vi "Arcade Drive.vi"(8 "b":dbl=1.0, 9 "a":dbl=1.0, 11 "Drive Metrics In":T1) -> (3 "Drive Metrics out":T1)   [LabVIEW 2014]
uses:
  Drive Train Metrics.ctl
  CmdFlag.ctl
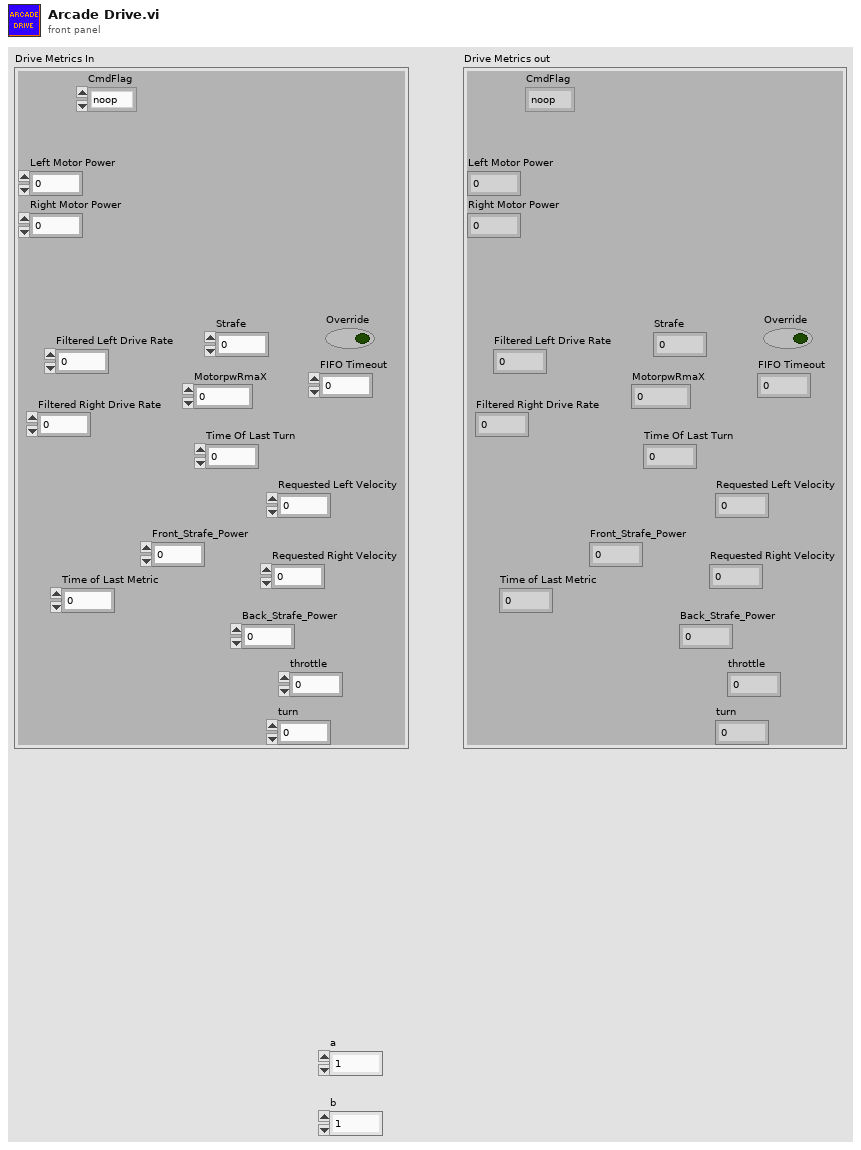
[diagram p1: front panel]
types:
  T1 = typedef "Drive Train Metrics.ctl" = cluster{"CmdFlag":T2, "Right Motor Power":dbl, "Left Motor Power":dbl, "Filtered Left Drive Rate":dbl, "Filtered Right Drive Rate":dbl, "Time of Last Metric":u32, "FIFO Timeout":i32, "Requested Left Velocity":dbl, "Requested Right Velocity":dbl, "throttle":dbl, "turn":dbl, "MotorpwRmaX":i32, "Strafe":dbl, "Override":bool, "Time Of Last Turn":dbl, "Front_Strafe_Power":dbl, "Back_Strafe_Power":dbl}
  T2 = typedef "CmdFlag.ctl" = enum16{"noop", "suspend", "resume"}
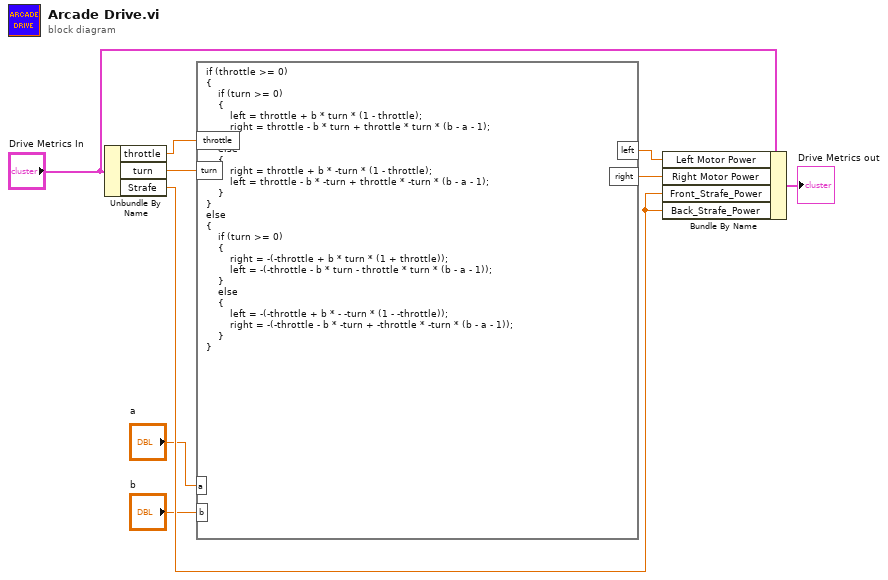
[diagram p0: block diagram]
diagram:
  n1 = Unbundle By Name("Drive Metrics In") -> ("throttle"=w5:dbl, "turn"=w4:dbl, "Strafe"=w8:dbl)
  n2 = formula code="if (throttle >= 0)\n{\n    if (turn >= 0)\n    {\n        left = throttle + b * turn * (1 - throttle);\n        right = throttle - b * turn + throttle * turn * (b - a - 1);\n    }\n    else\n    {\n        right = throttle + b * -turn * (1 - throttle);\n        left = throttle - b * -turn + throttle * -turn * (b - a - 1);\n    }\n}\nelse\n{\n    if (turn >= 0)\n    {\n        right = -(-throttle + b * turn * (1 + throttle));\n        left = -(-throttle - b * turn - throttle * turn * (b - a - 1));\n    }\n    else\n    {\n        left = -(-throttle + b * - -turn * (1 - -throttle));\n        right = -(-throttle - b * -turn + -throttle * -turn * (b - a - 1));\n    }\n}"("throttle"=w5, "turn"=w4, "a"="a", "b"="b") -> ("left"=w3:dbl, "right"=w2:dbl)
  n3 = Bundle By Name(cluster="Drive Metrics In", "Left Motor Power"=w3, "Right Motor Power"=w2, "Front_Strafe_Power"=w8, "Back_Strafe_Power"=w8) -> (→"Drive Metrics out":T1)
